vi "All Clients.vi"(8 "error in (no error)":errorcluster, 11 "Basic WebSocket Manager in":refnum<class "Basic WebSocket Manager.lvclass">) -> (0 "error out":errorcluster, 2 "Clients":refnum<class "WebSocket Client.lvclass">[](array[class]), 3 "Basic WebSocket Manager out":refnum<class "Basic WebSocket Manager.lvclass">)   [LabVIEW 2020, in "HTTP Server.lvlib" / "Basic WebSocket Manager.lvclass"]
uses:
  Basic WebSocket Manager.lvclass
  Basic WebSocket Manager.lvclass/Basic WebSocket Manager.ctl
  WebSocket Client/WebSocket Client.lvclass
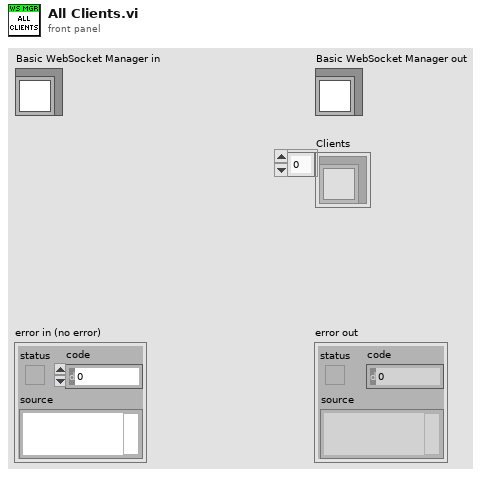
[diagram p1: front panel]
types:
  T1 = typedef "HTTP Server.lvlib/Basic WebSocket Manager.lvclass/Ref Data.ctl" = cluster{"Clients":map{string, refnum<class "WebSocket Client.lvclass">}}
  T2 = map{string, refnum<class "WebSocket Client.lvclass">}
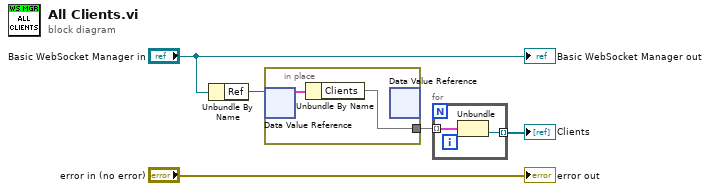
[diagram p0: block diagram]
diagram:
  n1 = Unbundle By Name("Basic WebSocket Manager in") -> ("Ref"=w4:refnum<data-value>)
  n2 = in-place {
    in-place-border: [w6] -> w2
    n3 = in-place-dvr #1(w4) -> (w7:T1)  [unwired: 1 out]
    n4 = Unbundle By Name(w7) -> ("Clients"=w6:T2)
    n5 = in-place-dvr #1() -> ()  [unwired: 1 in, 2 out]
  }
  n6 = for {
    tunnel: [w9] -> w1 mode=indexing
    tunnel: w2 -> [w8] mode=indexing
    n7 = Unbundle(w8) -> ("Client"=w9:refnum<class "WebSocket Client.lvclass">)  [unwired: 1 out]
  }
  "Clients" <- w1
  "error out" <- "error in (no error)"
  "Basic WebSocket Manager out" <- "Basic WebSocket Manager in"
